vi "OAT Tachless Update Chkpoints (Auto Place).vi"(4 "Update Cursor":bool, 5 "RefNum":T1, 6 "sampling frequency [Hz]":dbl=1.0 format="%.2f", 7 "XY Max Range":T2 {"YScale.Range"."Start" format="%.2f"; "YScale.Range"."Minor Incr" format="%.2f"; "YScale.Range"."Increment" format="%.2f"; "YScale.Range"."Maximum" format="%.2f"; "YScale.Range"."Minimum" format="%.2f"; "XScale.Range"."Start" format="%.2f"; "XScale.Range"."Minor Incr" format="%.2f"; "XScale.Range"."Increment" format="%.2f"; "XScale.Range"."Maximum" format="%.2f"; "XScale.Range"."Minimum" format="%.2f"}, 9 "chkpoint color":u32(colorbox)=15593216, 11 "Tracks ref":refnum<vi>) -> (1 "Boundary":cluster{"X":dbl[], "Y":dbl[]} {"Y" format="%.2f"; "X" format="%.2f"}, 2 "ChkPoints":cluster{"X":dbl[], "Y":dbl[]} {"Y" format="%.2f"; "X" format="%.2f"})   [LabVIEW 2017, in "SoundVib_Tachless.lvlib"]
uses:
  <vilib>/addons/Sound and Vibration/Order Analysis/Tachless/SoundVib_Tachless.lvlib
  <vilib>/addons/Sound and Vibration/Order Analysis/Ref Gabor Order Tracking/GT RefNum.ctl
  <vilib>/addons/Sound and Vibration/Order Analysis/Gabor Order Tracking/SoundVib_Gabor.lvlib
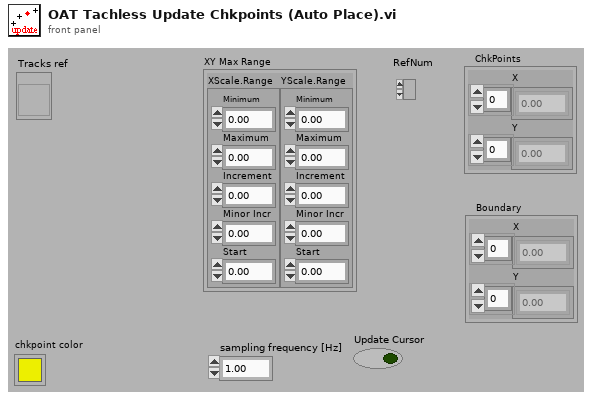
[diagram p1: front panel]
types:
  T1 = typedef "SoundVib_Gabor.lvlib/GT RefNum.ctl" = refnum<k1>
  T2 = cluster{"XScale.Range":cluster{"Minimum":dbl, "Maximum":dbl, "Increment":dbl, "Minor Incr":dbl, "Start":dbl}, "YScale.Range":cluster{"Minimum":dbl, "Maximum":dbl, "Increment":dbl, "Minor Incr":dbl, "Start":dbl}}
  T3 = cluster{"Name":string, "Color":u32, "Style":u8, "Point Style":u8, "Name Visible":bool, "Allow Drag":bool, "Lock Style":u32, "Plot":u32, "Index":i32, "Position":cluster{"X":dbl, "Y":dbl}}[]
  T4 = cluster{"Name":string, "Color":u32, "Hair Style":u8, "Point Style":u8, "Name Visible":bool, "Trackable":bool, "Lock Style":u32, "Plot Number":u32, "Marker Index":i32, "Location":cluster{"X":dbl, "Y":dbl}}[]
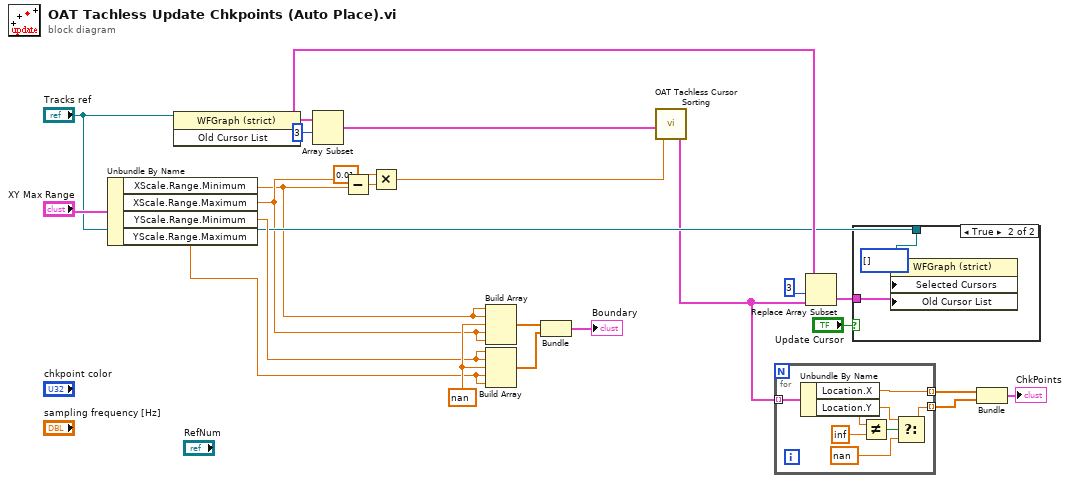
[diagram p0: block diagram]
diagram:
  w21 = nan
  n1 = Unbundle By Name("XY Max Range") -> ("XScale.Range.Minimum"=w8:dbl, "XScale.Range.Maximum"=w9:dbl, "YScale.Range.Minimum"=w17:dbl, "YScale.Range.Maximum"=w16:dbl)
  n2 = property on="Property Node" class="WFGraph (strict)"(reference="Tracks ref") -> ("Old Cursor List"=w12:T3)  [unwired: 1 in, 2 out]
  n3 = Array Subset(array=w12, index=3 ("Array Index")) -> (w2:T3)  [unwired: 1 in]
  n4 = Subtract(x=w9, y=w8) -> (x-y=w7:dbl)
  n5 = Multiply(x=0.01, y=w7) -> (x*y=w5:dbl)
  n6 = Build Array(w8, w8, w21, w9, w9) -> (w20:dbl[])
  n7 = Build Array(w17, w17, w21, w16, w16) -> (w19:dbl[])
  n8 = Bundle(w20, w19) -> (→"Boundary":cluster{dbl[], dbl[]})  [unwired: 1 in]
  n9 = call <vilib>:"OAT Tachless Cursor Sorting.vi"("Numeric"=w5, "Array"=w2) -> ("Array 2"=w3:T4)
  n10 = for {
    tunnel: w3 -> [w30] mode=indexing
    tunnel: [w29] -> w15 mode=indexing
    tunnel: [w24] -> w14 mode=indexing
    n11 = Unbundle By Name(w30) -> ("Location.X"=w29:dbl, "Location.Y"=w26:dbl)
    n12 = Not Equal?(x=w26, y=inf) -> (x != y?=w27:bool)
    n13 = Select(t=w26, s=w27, f=nan) -> (s? t:f=w24:dbl)
  }
  n14 = Replace Array Subset(array=w12, new element=w3, index=3 ("Index")) -> (w4:T3)
  n15 = case shown="True" "Update Cursor" {
    tunnel: "Tracks ref" -> [_ w33]
    tunnel: w4 -> [_ w32]
    frame False {
    }
    frame True {
      n16 = property on="Property Node" class="WFGraph (strict)"(reference=w33, "Selected Cursors"=u32[] [], "Old Cursor List"=w32) -> ()  [unwired: 1 in, 2 out]
    }
  }
  n17 = Bundle(w15, w14) -> (→"ChkPoints":cluster{dbl[], dbl[]})  [unwired: 1 in]
